vi "Main.vi"() -> ()   [LabVIEW 2020]
panel:
  out "String":string
  in  "Boolean":bool
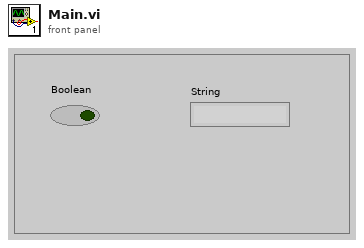
[diagram p1: front panel]
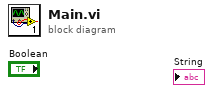
[diagram p0: block diagram]
diagram:
